vi "2D Quadrature (VI).vi"(7 "data":variant, 8 "tolerance":dbl=1e-05, 9 "Lower Limits":T1, 10 "Upper Limits":T2={"x upper limit"=1.0, "y upper limit"=1.0}, 11 "integrand":refnum<vi>) -> (0 "error":i32, 3 "result":dbl)   [LabVIEW 2020, in "NI_AALPro.lvlib"]
doc: "Performs numerical integration using adaptive quadrature approach. You must manually select the polymorphic instance to use."
uses:
  <vilib>/Analysis/NI_AALPro.lvlib
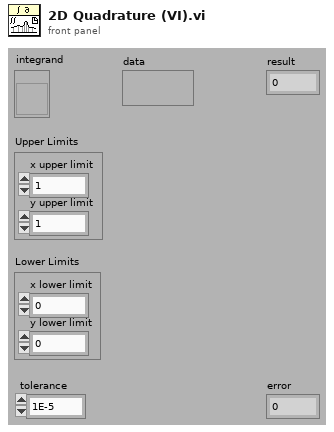
[diagram p1: front panel]
types:
  T1 = cluster{"x lower limit":dbl, "y lower limit":dbl}
  T2 = cluster{"x upper limit":dbl, "y upper limit":dbl}
  T3 = cluster{"x lower limit":dbl, "x upper limit":dbl}
  T4 = cluster{"y lower limit":dbl, "y upper limit":dbl}
  T5 = cluster{cluster{"x lower limit":dbl, "x upper limit":dbl}, cluster{"y lower limit":dbl, "y upper limit":dbl}}
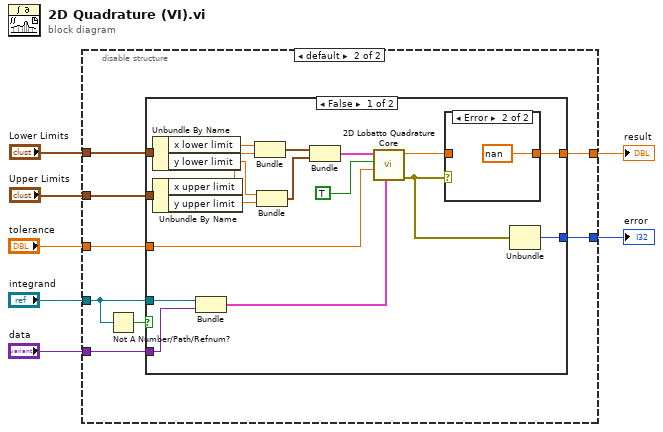
[diagram p0: block diagram]
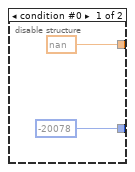
[diagram p2: hidden frame]
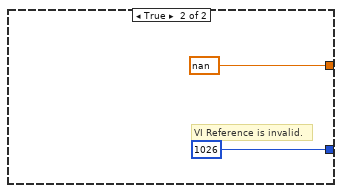
[diagram p4: hidden frame]
diagram:
  n1 = disable-structure shown="default" {
    disable-tunnel: [-20078 ("code") w17] -> w7
    disable-tunnel: "Upper Limits" -> [_ w16]
    disable-tunnel: "Lower Limits" -> [_ w15]
    disable-tunnel: "tolerance" -> [_ w14]
    disable-tunnel: [nan ("result") w13] -> w5
    disable-tunnel: "integrand" -> [_ w11]
    disable-tunnel: "data" -> [_ w10]
    frame condition #0 {
    }
    frame condition #1 (active) {
      n2 = Not A Number/Path/Refnum?(number/path/refnum=w11) -> (NaN/Path/Refnum?=w12:bool)
      n3 = case shown="False" w12 {
        tunnel: [w35 nan] -> w13
        tunnel: [w34 1026] -> w17
        tunnel: w16 -> [w31 _]
        tunnel: w15 -> [w30 _]
        tunnel: w14 -> [w18 _]
        tunnel: w11 -> [w23 _]
        tunnel: w10 -> [w22 _]
        frame False {
          n4 = Unbundle By Name(w30) -> ("x lower limit"=w29:dbl, "y lower limit"=w25:dbl)
          n5 = Unbundle By Name(w31) -> ("x upper limit"=w28:dbl, "y upper limit"=w26:dbl)
          n6 = Bundle("integrand"=w23, "data"=w22) -> (w21:cluster{"integrand":refnum<vi>, "data":variant})  [unwired: 1 out]
          n7 = Bundle("x lower limit"=w29, "x upper limit"=w28) -> (w27:T3)  [unwired: 1 out]
          n8 = Bundle("y lower limit"=w25, "y upper limit"=w26) -> (w24:T4)  [unwired: 1 out]
          n9 = Bundle(w27, w24) -> (w20:T5)  [unwired: 1 out]
          n10 = call <vilib>:"2D Lobatto Quadrature Core.vi"("VI ref"=w21, "tolerance"=w18, "Formula/VI ref"=TRUE, "limits"=w20) -> ("error out"=w32:errorcluster, "result"=w33:dbl)  [unwired: 2 in, 4 out]
          n11 = case shown="Error" w32 {
            tunnel: w33 -> [w36 _]
            tunnel: [w36 nan] -> w35
            frame No Error {
            }
            frame Error {
            }
          }
          n12 = Unbundle(w32) -> ("code"=w34:i32)  [unwired: 2 out]
        }
        frame True {
          # "VI Reference is invalid."
        }
      }
    }
  }
  "error" <- w7
  "result" <- w5
